vi "Configure Generator Tracking.vi"(4 "Phase Relationship (0 Degrees)":i32, 5 "Enable Frequency Tracking (F: Disable)":bool, 6 "Copy Signal (F: Disable)":bool, 7 "Enable Amplitude Tracking (F: Disable)":bool, 8 "error in (no error)":errorcluster, 9 "Enable Tracking (F: Disable)":bool, 10 "Waveform Generator Number (1: Waveform Generator 1)":i32(ring)=1 items=["Waveform Generator 1"=1, "Waveform Generator 2"=2], 11 "VISA resource name":refnum<visa-resource-name>) -> (0 "error out":errorcluster, 3 "VISA resource name out":refnum<visa-resource-name>)   [LabVIEW 2016, in "Agilent 2000 3000 X-Series.lvlib"]
doc: "Configures waveform generator tracking.\n\n<b>Note:</b>\nOnly supported for the 4000x series models"
uses:
  Agilent 2000 3000 X-Series.lvlib
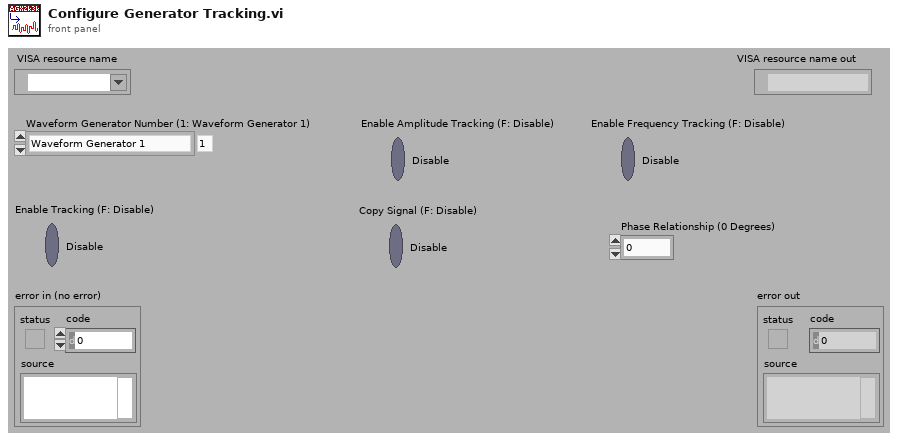
[diagram p1: front panel]
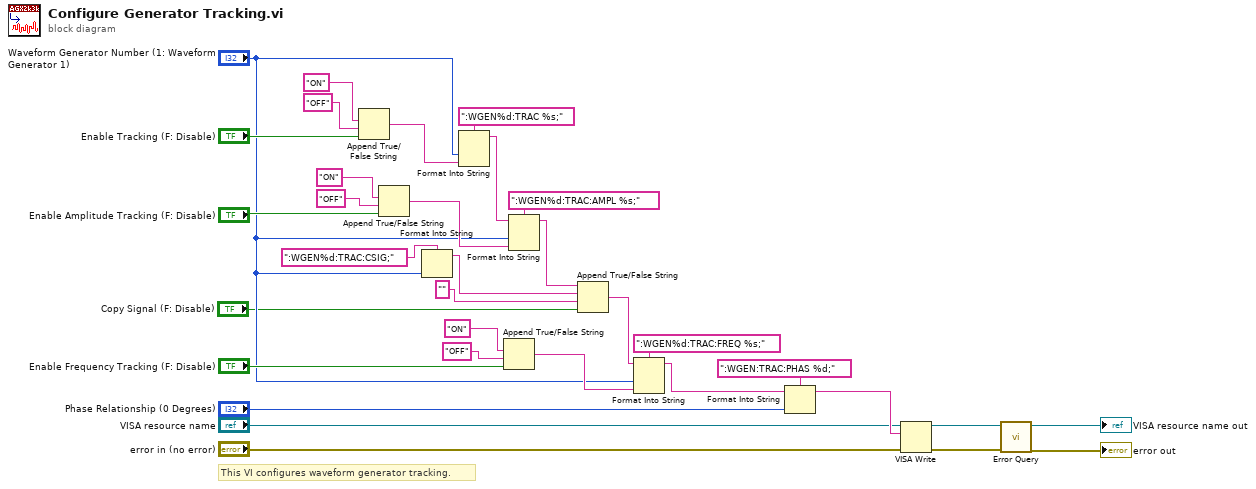
[diagram p0: block diagram]
diagram:
  # "This VI configures waveform generator tracking."
  n1 = Append True/False String(1:"Enable Tracking (F: Disable)", 2:"OFF", 3:"ON") -> (0:w29:string)  [unwired: 1 out]
  n2 = Append True/False String(1:"Enable Amplitude Tracking (F: Disable)", 2:"OFF", 3:"ON") -> (0:w23:string)  [unwired: 1 out]
  n3 = Format Into String(format string=":WGEN%d:TRAC:CSIG;", "Waveform Generator Number (1: Waveform Generator 1)") -> (resulting string=w11:string)  [unwired: 2 in, 1 out]
  n4 = Format Into String(format string=":WGEN%d:TRAC %s;", "Waveform Generator Number (1: Waveform Generator 1)", w29) -> (resulting string=w25:string)  [unwired: 2 in, 1 out]
  n5 = Append True/False String(1:"Enable Frequency Tracking (F: Disable)", 2:"OFF", 3:"ON") -> (0:w18:string)  [unwired: 1 out]
  n6 = Format Into String(format string=":WGEN%d:TRAC:AMPL %s;", initial string=w25, "Waveform Generator Number (1: Waveform Generator 1)", w23) -> (resulting string=w7:string)  [unwired: 1 in, 1 out]
  n7 = Append True/False String(1:"Copy Signal (F: Disable)", 2:"", 3:w11, 4:w7) -> (0:w8:string)
  n8 = Format Into String(format string=":WGEN%d:TRAC:FREQ %s;", initial string=w8, "Waveform Generator Number (1: Waveform Generator 1)", w18) -> (resulting string=w6:string)  [unwired: 1 in, 1 out]
  n9 = Format Into String(format string=":WGEN:TRAC:PHAS %d;", initial string=w6, "Phase Relationship (0 Degrees)") -> (resulting string=w5:string)  [unwired: 1 in, 1 out]
  n10 = VISA Write(VISA resource name="VISA resource name", write buffer=w5, error in (no error)="error in (no error)") -> (VISA resource name out=w17:refnum<visa-resource-name>, error out=w16:errorcluster)  [unwired: 1 out]
  n11 = call "Error Query.vi"("error in (no error)"=w16, "VISA resource name"=w17) -> ("error out"=→"error out":errorcluster, "VISA resource name out"=→"VISA resource name out":refnum<visa-resource-name>)  [unwired: 8 out]
